vi "判定取舍.vi"(0 "判定 1":string[][](table)=[["235", "2342", "32432"], ["32432", "324", "324"], ["", "234", "32432"]], 3 "判定 2":string[][](table)=[["", ""], ["", ""]]) -> (2 "判定 3":string[][](array[string]))   [LabVIEW 2019]
panel:
  in  "布尔":bool
  out "元素":i32
  out "数值":i32
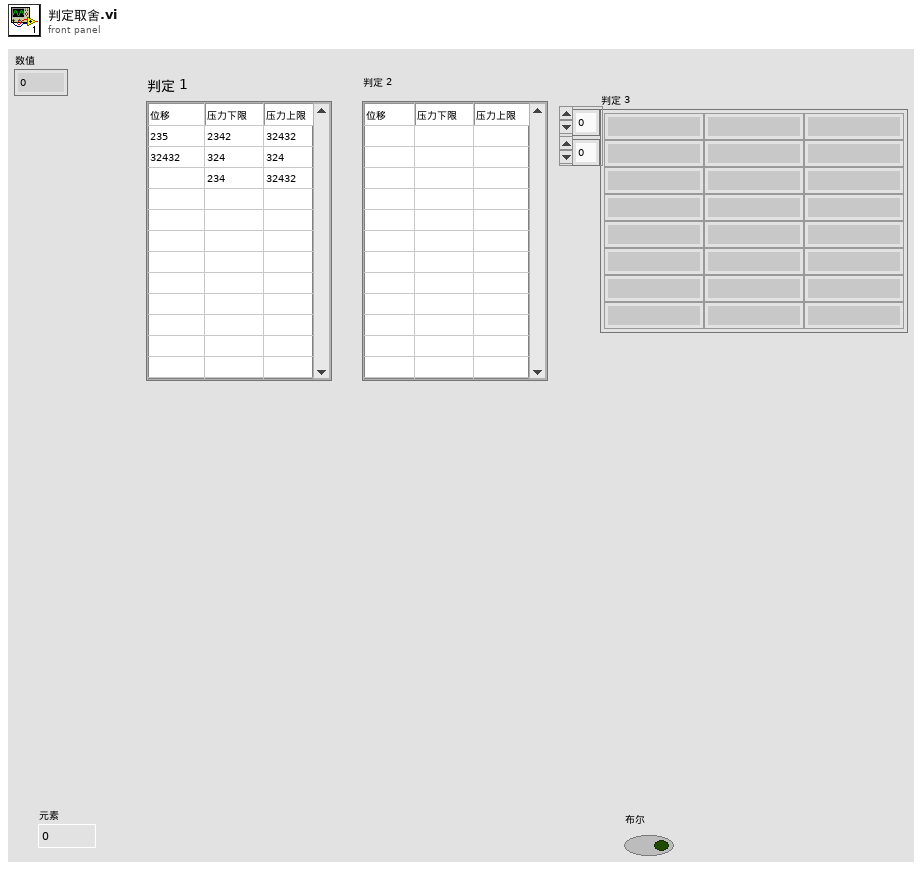
[diagram p1: front panel]
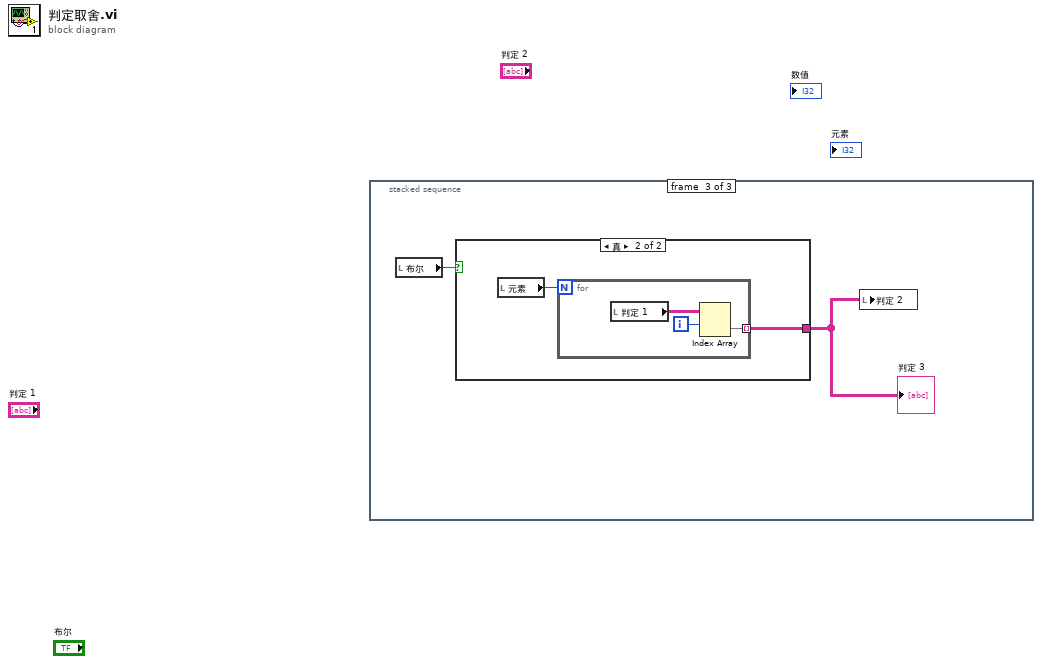
[diagram p0: block diagram]
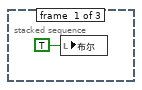
[diagram p2: hidden frame]
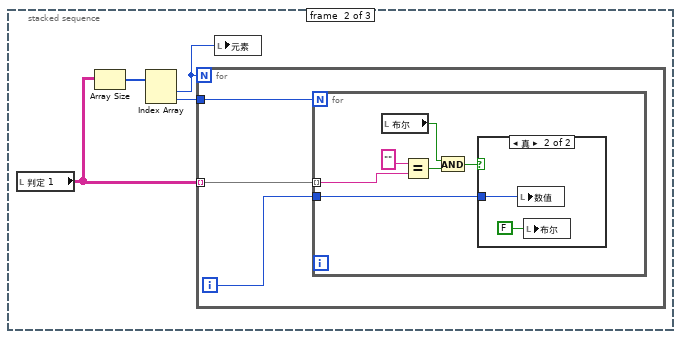
[diagram p3: hidden frame]
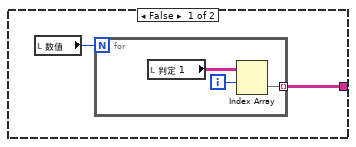
[diagram p5: hidden frame]
diagram:
  n1 = stacked-sequence {
    frame #0 {
      n2 = local write "布尔"(TRUE ("布尔")) -> ()
    }
    frame #1 {
      n3 = local read "判定 1"() -> (w4:string[][])
      n4 = Array Size(array=w4) -> (size(s)=w3:i32[])
      n5 = Index Array(array=w3) -> (element #1=w2:i32, element #2=w5:i32)  [unwired: 2 in]
      n6 = for {
        N: w2 -> [_]
        tunnel: w5 -> [w8]
        tunnel: w4 -> [w7] mode=indexing
        i -> [w6]
        n7 = for {
          N: w8 -> [_]
          tunnel: w7 -> [w13] mode=indexing
          tunnel: w6 -> [w12]
          n8 = local read "布尔"() -> (w10:bool)
          n9 = Equal?(x="", y=w13) -> (x = y?=w11:bool)
          n10 = And(x=w10, y=w11) -> (x .and. y?=w9:bool)
          n11 = case shown="真" w9 {
            tunnel: w12 -> [_ w15]
            frame False {
            }
            frame True {
              n12 = local write "数值"(w15) -> ()
              n13 = local write "布尔"(FALSE ("布尔")) -> ()
            }
          }
        }
      }
      n14 = local write "元素"(w2) -> ()
    }
    frame #2 {
      n15 = local read "布尔"() -> (w18:bool)
      n16 = case shown="真" w18 {
        tunnel: [w19 w25] -> w17
        frame False {
          n17 = local read "数值"() -> (w20:i32)
          n18 = for {
            N: w20 -> [_]
            tunnel: [w21] -> w19 mode=indexing
            i -> [w22]
            n19 = local read "判定 1"() -> (w23:string[][])
            n20 = Index Array(array=w23, index (row)=w22) -> (element=w21:string[])  [unwired: 1 in]
          }
        }
        frame True {
          n21 = local read "元素"() -> (w24:i32)
          n22 = for {
            N: w24 -> [_]
            tunnel: [w26] -> w25 mode=indexing
            i -> [w27]
            n23 = local read "判定 1"() -> (w28:string[][])
            n24 = Index Array(array=w28, index (row)=w27) -> (element=w26:string[])  [unwired: 1 in]
          }
        }
      }
      "判定 3" <- w17
      n25 = local write "判定 2"(w17) -> ()
    }
  }
